vi "From Variant.vi"(8 "error in (no error)":errorcluster, 10 "Variant":variant) -> (0 "error out":errorcluster, 3 "JSON Array out":refnum<class "JSON Datatype.lvclass">)   [LabVIEW 2015, in "LVJSON.lvlib" / "JSON Datatype.lvclass"]
uses:
  JSON Data Classes/JSON Datatype/JSON Datatype.lvclass
  JSON Data Classes/JSON Numeric/JSON Numeric.lvclass
  JSON Data Classes/JSON String/JSON String.lvclass
  JSON Data Classes/JSON Boolean/JSON Boolean.lvclass
  JSON Data Classes/JSON Array/JSON Array.lvclass
  JSON Data Classes/JSON Object/JSON Object.lvclass
  JSON Data Classes/JSON Null/JSON Null.lvclass
  JSON Data Classes/JSON String/New JSON String.vi
  <vilib>/Utility/Data Type/NI_Data Type.lvlib
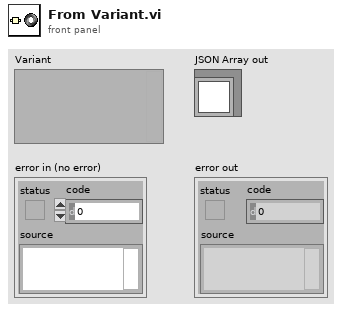
[diagram p1: front panel]
types:
  T1 = typedef "NI_Data Type.lvlib/Data Type.ctl" = enum8{"Invalid Type", "Void", "I8", "I16", "I32", "I64", "U8", "U16", "U32", "U64", "Single Float", "Double Float", "Extended Float", "Single Complex", "Double Complex", "Extended Complex", "Enum U8", "Enum U16", "Enum U32", "Enum U64", "Single Float With Unit", "Double Float With Unit", "Extended Float With Unit", "Single Complex with Unit", "Double Complex with Unit", "Extended Complex with Unit", "Boolean", "String", "Path", "Picture", "Tag", "Array", "Cluster", "Variant", "LV Variant", "Waveform", "Timestamp", "Digital Waveform", "Digital Data", "ExpressData", "Refnum", "External Data", "VI", "Poly VI", "LabVIEW Class Instance", "Fixed Point"}
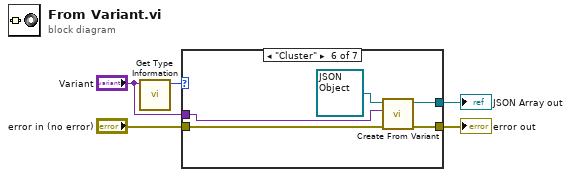
[diagram p0: block diagram]
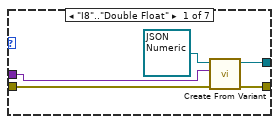
[diagram p2: hidden frame]
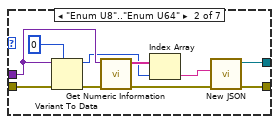
[diagram p3: hidden frame]
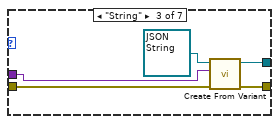
[diagram p4: hidden frame]
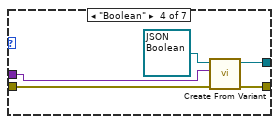
[diagram p5: hidden frame]
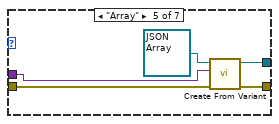
[diagram p6: hidden frame]
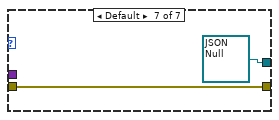
[diagram p7: hidden frame]
diagram:
  n1 = call <vilib>:"Get Type Information.vi"("Variant"="Variant") -> ("Type"=w5:T1)  [unwired: 6 in, 4 out]
  n2 = case shown="\"Cluster\"" w5 {
    tunnel: "Variant" -> [w9 w18 w24 w29 w34 w39 _]
    tunnel: [w6 w20 w21 w26 w33 w36 refnum<class "JSON Null.lvclass"> refnum ("JSON String out")] -> w1
    tunnel: "error in (no error)" -> [w8 w13 w23 w28 w32 w38 w41]
    tunnel: [w7 w19 w22 w27 w31 w37 w41] -> w2
    frame "I8".."Double Float" {
      n3 = call-dynamic "Create From Variant.vi"("error in (no error)"=w8, "Variant"=w9, "JSON Numeric in"=refnum<class "JSON Numeric.lvclass"> refnum ("JSON Object in")) -> ("error out"=w7:errorcluster, "JSON Numeric out"=w6:refnum<class "JSON Numeric.lvclass">)  [unwired: 7 in]
    }
    frame "Enum U8".."Enum U64" {
      n4 = Variant To Data(error in=w13, type=u64 0, Variant=w18) -> (data=w15:u64, error out=w12:errorcluster)
      n5 = call <vilib>:"Get Numeric Information.vi"("error in (no error)"=w12, "Variant"=w18) -> ("error out"=w11:errorcluster, "Enum Names"=w16:string[])  [unwired: 6 in, 2 out]
      n6 = Index Array(array=w16, index=w15) -> (element=w14:string)
      n7 = call-poly "New JSON.vi"("error in (no error)"=w11, "value"=w14) -> ("error out"=w19:errorcluster, "JSON String out"=w20:refnum<class "JSON String.lvclass">)  [unwired: 8 in]
    }
    frame "String" {
      n8 = call-dynamic "Create From Variant.vi"("error in (no error)"=w23, "Variant"=w24, "JSON String in"=refnum<class "JSON String.lvclass"> refnum ("JSON Object in")) -> ("error out"=w22:errorcluster, "JSON String out"=w21:refnum<class "JSON String.lvclass">)  [unwired: 7 in]
    }
    frame "Boolean" {
      n9 = call-dynamic "Create From Variant.vi"("error in (no error)"=w28, "Variant"=w29, "JSON Boolean in"=refnum<class "JSON Boolean.lvclass"> refnum ("JSON Object in")) -> ("error out"=w27:errorcluster, "JSON Boolean out"=w26:refnum<class "JSON Boolean.lvclass">)  [unwired: 7 in]
    }
    frame "Array" {
      n10 = call-dynamic "Create From Variant.vi"("error in (no error)"=w32, "Variant"=w34, "JSON Array in"=refnum<class "JSON Array.lvclass"> refnum ("JSON Object in")) -> ("error out"=w31:errorcluster, "JSON Array out"=w33:refnum<class "JSON Array.lvclass">)  [unwired: 7 in]
    }
    frame "Cluster" {
      n11 = call-dynamic "Create From Variant.vi"("error in (no error)"=w38, "Variant"=w39, "JSON Object in"=refnum<class "JSON Object.lvclass"> refnum) -> ("error out"=w37:errorcluster, "JSON Object out"=w36:refnum<class "JSON Object.lvclass">)  [unwired: 7 in]
    }
    frame Default {
    }
  }
  "error out" <- w2
  "JSON Array out" <- w1
